vi "KnrEncoderTest.vi"() -> ()   [LabVIEW 2019]
uses:
  <vilib>/Platform/TimedLoop/XDataNode/timing_clust.ctl
  <vilib>/Platform/TimedLoop/XDataNode/nitl_modes.ctl
  <vilib>/Platform/TimedLoop/XDataNode/wakeup.ctl
  KNRm_ReMi_OS5.lvlibp/KNRm_ReMi_Toolkit/IO/LowLevel/IO_Channel_DIO.ctl
  KNRm_ReMi_OS5.lvlibp/KNRm_ReMi_Toolkit/IO/LowLevel/IO_Channel_Motor.ctl
  <vilib>/Platform/TimedLoop/XDataNode/XDataNode.xnode
  <vilib>/Platform/TimedLoop/XDataNode/XDNodeRunTimeDep.lvlib
  KNRm_ReMi_OS5.lvlibp
panel:
  in  "4xMotorSpeed(PWM%)":dbl[](array[numeric])=[0.0, 0.0, 0.0, 0.0]
  in  "Reset 2":bool
  out "ENC 3":i32
  out "ENC 4":i32
  in  "stop":bool
  out "error out":errorcluster
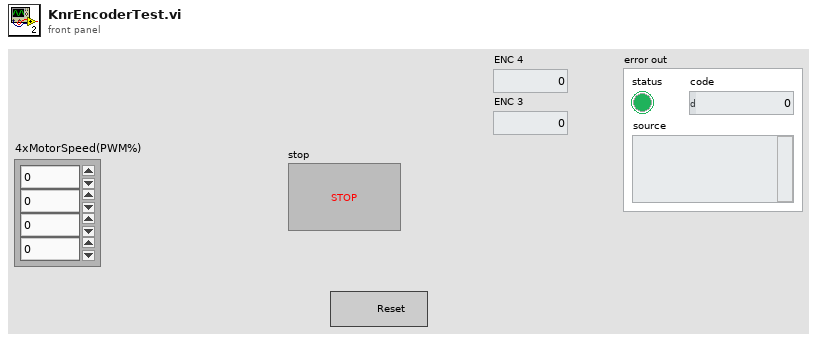
[diagram p1: front panel]
types:
  T1 = typedef "KNRm_ReMi_OS5.lvlibp/IO_Channel_DIO.ctl" = enum16{"B/DIO1 (M1)", "A/DIO8 (M2)", "B/DIO7 (M3)", "A/DIO3 (M4)", "A/DIO14 (RC1_0)", "A/DIO15 (RC1_1)"}
  T2 = typedef "XDNodeRunTimeDep.lvlib/timing_clust.ctl" = cluster{"Expected End [f-1]":u64, "Actual End [f-1]":u64, "Finished Late? [f-1]":bool, "Expected End [i-1]":u64, "Actual End [i-1]":u64, "Finished Late? [i-1]":bool, "Expected Start [i]":u64, "Actual Start [i]":u64, "Expected Start [f]":u64, "Actual Start [f]":u64, "Source Name":string, "Structure Name":string, "Period":i64, "Deadline":i64, "Offset":i64, "Start":i64, "Priority":i32, "Timeout":i32, "Mode":T3, "Wakeup Reason":T4, "Error":errorcluster, "Source Type":string, "Secondary Source Type":string, "Global End Time":u64, "Global Start Time":u64, "Frame Duration":u64, "Iteration Duration":u64, "Assigned CPU":i32, "I/O Scan Engine Mode":u32}
  T3 = typedef "XDNodeRunTimeDep.lvlib/nitl_modes.ctl" = enum32{"No Change", "Process missed periods, maintain original phase", "Discard missed periods, maintain original phase", "Process missed periods, ignore original phase", "Discard missed periods, ignore original phase"}
  T4 = typedef "XDNodeRunTimeDep.lvlib/wakeup.ctl" = enum32{"Normal", "Aborted", "Asynchronous wakeup", "Timing source error", "Timed loop error", "Timeout"}
  T5 = typedef "KNRm_ReMi_OS5.lvlibp/IO_Channel_Motor.ctl" = enum16{"M1", "M2", "M3", "M4"}
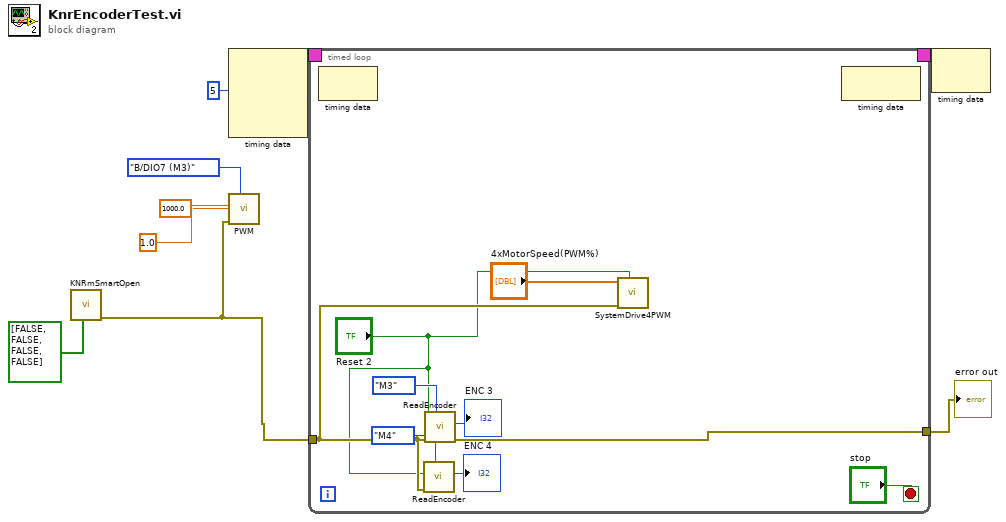
[diagram p0: block diagram]
diagram:
  n1 = call "KNRmSmartOpen.vi"("SpeedMode"=bool[] [FALSE, FALSE, FALSE, FALSE]) -> ("error out"=w1:errorcluster)  [unwired: 8 in, 2 out]
  n2 = node-c288(i64 5 ("Period")) -> (w9:T2)  [unwired: 3 in]
  n3 = call "PWM.vi"("IO_Chanel"=IO_Channel_DIO."B/DIO7 (M3)", "error in"=w1, "DutyCycle"=1.0, "Frequency(Hz)"=1000.0) -> ()  [unwired: 7 in, 1 out]
  n4 = timed-loop {
    timing: w9 -> [_]
    timing-out: [_] -> w8
    tunnel: [w15] -> w6
    tunnel: w1 -> [w12]
    stop <- "stop" stop-if-true
    n5 = node-c288() -> ()  [unwired: 1 in, 1 out]
    n6 = call "ReadEncoder.vi"("Channel"=IO_Channel_Motor."M4", "error in"=w12, "Reset"="Reset 2") -> ("ENC (count)"=→"ENC 4":i32)  [unwired: 7 in, 1 out]
    n7 = call "ReadEncoder.vi"("Channel"=IO_Channel_Motor."M3", "error in"=w12, "Reset"="Reset 2") -> ("error out"=w15:errorcluster, "ENC (count)"=→"ENC 3":i32)  [unwired: 7 in]
    n8 = call "SystemDrive4PWM.vi"("Reset"="Reset 2", "error in"=w12, "4xMotorSpeed(PWM%)"="4xMotorSpeed(PWM%)") -> ()  [unwired: 7 in, 2 out]
    n9 = node-c288() -> ()  [unwired: 1 in, 1 out]
  }
  "error out" <- w6
  n10 = node-c288(w8) -> ()  [unwired: 1 out]
